vi "Pre Launch Init.vi"(11 "MuxActor in":refnum<class "MuxActor.lvclass">) -> (0 "error out":errorcluster, 3 "MuxActor out":refnum<class "MuxActor.lvclass">)   [LabVIEW 2022 SP3, in "VideoMux.lvlib" / "MuxActor.lvclass"]
doc: "(<B>Filename</B>: Actor Framework.lvlib:Actor.lvclass:Pre Launch Init.vi)\n\nDefines behavior that occurs after the Launch Actor method is invoked but before the actor's Actor Core method begins running.\n\nThe Pre Launch Init method is guaranteed to finish before the Launch Actor method returns to its caller and before the actor itself receives any messages. Any references that the Pre Launch Init method obtains are guaranteed to have the same lifetime as the actor itself. Any errors that the Pre Launch Init method returns will abort the launch.\n\nBy default, this method does nothing. A descendant class may override it to define behavior."
uses:
  MuxActor.lvclass
  MuxActor.lvclass/MuxActor.ctl
  <vilib>/IlluminatedG/IG Serial Stream/Stream-Serial/Serial Client/Serial Client.lvclass
  C:/Program Files (x86)/National Instruments/LabVIEW 2022/vi.lib/IlluminatedG/lv-stream/Connection/Connection.lvclass
  <vilib>/ActorFramework/Actor/Actor.lvclass
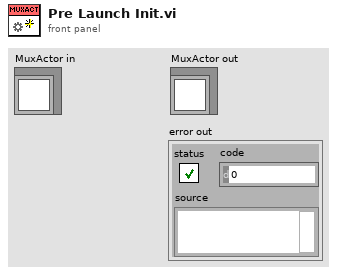
[diagram p1: front panel]
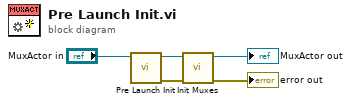
[diagram p0: block diagram]
diagram:
  n1 = call-parent "Pre Launch Init.vi"("Actor in"="MuxActor in") -> ("error out"=w2:errorcluster, "Actor out"=w4:refnum<class "MuxActor.lvclass">)  [unwired: 9 in]
  n2 = call "Init Muxes.vi"("error in (no error)"=w2, "MuxActor in"=w4) -> ("error out"=→"error out":errorcluster, "MuxActor out"=→"MuxActor out":refnum<class "MuxActor.lvclass">)  [unwired: 8 in]
